vi "Get Protocol List.vi"(8 "error in (no error)":errorcluster) -> (0 "error out":errorcluster, 3 "Class Lookup":variant)   [LabVIEW 2018, in "Protocols.lvlib"]
uses:
  Protocols.lvlib
  <vilib>/Utility/LVLibp/NI_PackedLibraryUtility.lvlib
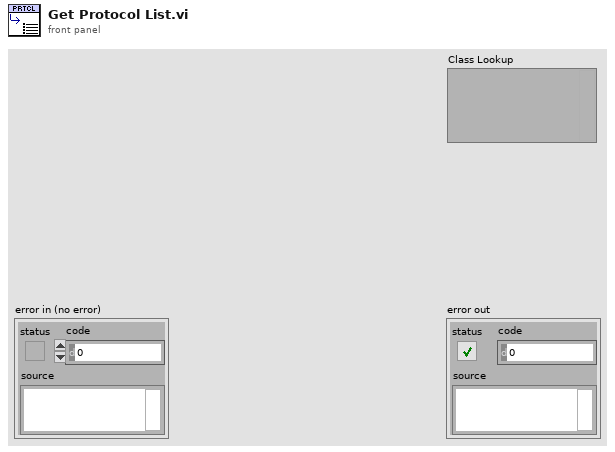
[diagram p1: front panel]
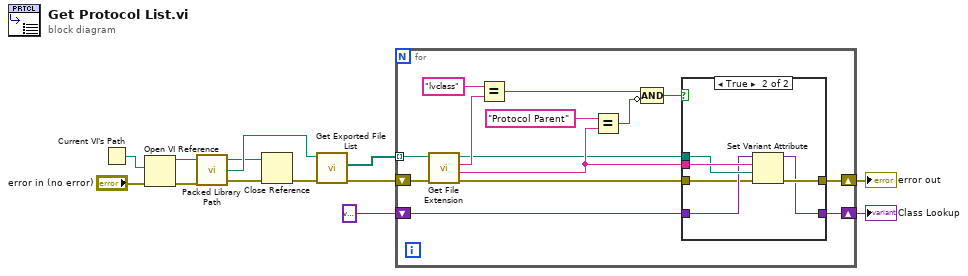
[diagram p0: block diagram]
diagram:
  n1 = Current VI's Path() -> (path=w8:path)
  n2 = Open VI Reference(vi path=w8, error in (no error)="error in (no error)") -> (vi reference=w7:refnum<vi>, error out=w4:errorcluster)  [unwired: 4 in]
  n3 = call <vilib>:"Packed Library Path.vi"("error in (no error)"=w4, "vi reference"=w7) -> ("error out"=w2:errorcluster, "packed library path"=w6:path, "vi reference out"=w5:refnum<vi>)  [unwired: 1 in]
  n4 = Close Reference(reference=w5, error in (no error)=w2) -> (error out=w1:errorcluster)
  n5 = call <vilib>:"Get Exported File List.vi"("error in (no error)"=w1, "packed library path"=w6) -> ("error out"=w12:errorcluster, "paths"=w13:path[])  [unwired: 7 in, 1 out]
  n6 = for {
    tunnel: w13 -> [w22] mode=indexing
    shift-right: [w16] -> w10
    shift-left: w12 -> [w23]
    shift-right: [w15] -> w9
    shift-left: variant ("variant") -> [w18]
    n7 = call <vilib>:"Get File Extension.vi"("error in (no error)"=w23, "file"=w22) -> ("error out"=w17:errorcluster, "filename without extension"=w20:string, "lowercase file extension"=w24:string, "dup file"=w19:path)  [unwired: 5 in, 1 out]
    n8 = Equal?(x="lvclass" ("string"), y=w24) -> (x = y?=w26:bool)
    n9 = Equal?(x="Protocol Parent", y=w20) -> (x = y?=w21:bool)
    n10 = Compound Arithmetic op=AND(w26, invert w21) -> (w14:bool)
    n11 = case shown="True" w14 {
      tunnel: w20 -> [_ w35]
      tunnel: w19 -> [_ w34]
      tunnel: w18 -> [w28 w33]
      tunnel: w17 -> [w29 w32]
      tunnel: [w29 w31] -> w16
      tunnel: [w28 w30] -> w15
      frame False {
      }
      frame True {
        n12 = Set Variant Attribute(Variant=w33, name=w35, value=w34, error in=w32) -> (Variant out=w30:variant, error out=w31:errorcluster)  [unwired: 1 out]
      }
    }
  }
  "error out" <- w10
  "Class Lookup" <- w9
